vi "rad_Configure Target Dialog.vi"(8 "Error In":errorcluster, 11 "Target Information in":T1={"Hostname"="", "Serial number"="", "Product name"="", "Product code"=0, "System status"="", "Credential type"=enum."None/Unlocked", "User added?"=FALSE, "Primary NIC"={"MAC address"="", "IP Address Request Mode"=2, "IP address"="", "Subnet mask"="", "Gateway"="", "DNS server"=""}, "System Credentials"={"Username"="", "Password"=""}} {"Primary NIC"."IP Address Request Mode" items=["Static"=1, "DHCP/Link-Local"=2, "Link-Local Only"=4, "DHCP Only"=8]}) -> (0 "Error Out":errorcluster, 3 "Target Information out":T1={"Hostname"="", "Serial number"="", "Product name"="", "Product code"=0, "System status"="", "Credential type"=enum."None/Unlocked", "User added?"=FALSE, "Primary NIC"={"MAC address"="", "IP Address Request Mode"=2, "IP address"="", "Subnet mask"="", "Gateway"="", "DNS server"=""}, "System Credentials"={"Username"="", "Password"=""}} {"Primary NIC"."IP Address Request Mode" items=["Static"=1, "DHCP/Link-Local"=2, "Link-Local Only"=4, "DHCP Only"=8]})   [LabVIEW 2020]
uses:
  support/SubVIs/Target Information.ctl
  TypeDefs/rad_Target Network Settings.ctl
  support/SubVIs/System Credentials.ctl
panel:
  in  "IP Address Request Mode":i32(ring)=2 items=["Static"=1, "DHCP/Link-Local"=2, "Link-Local Only"=4, "DHCP Only"=8]
  in  "DNS":string
  in  "Gateway":string
  in  "Subnet Mask":string
  in  "IP Address":string
  in  "Host Name":string
  in  "Cancel":bool
  in  "OK":bool
  # "Network Configuration"
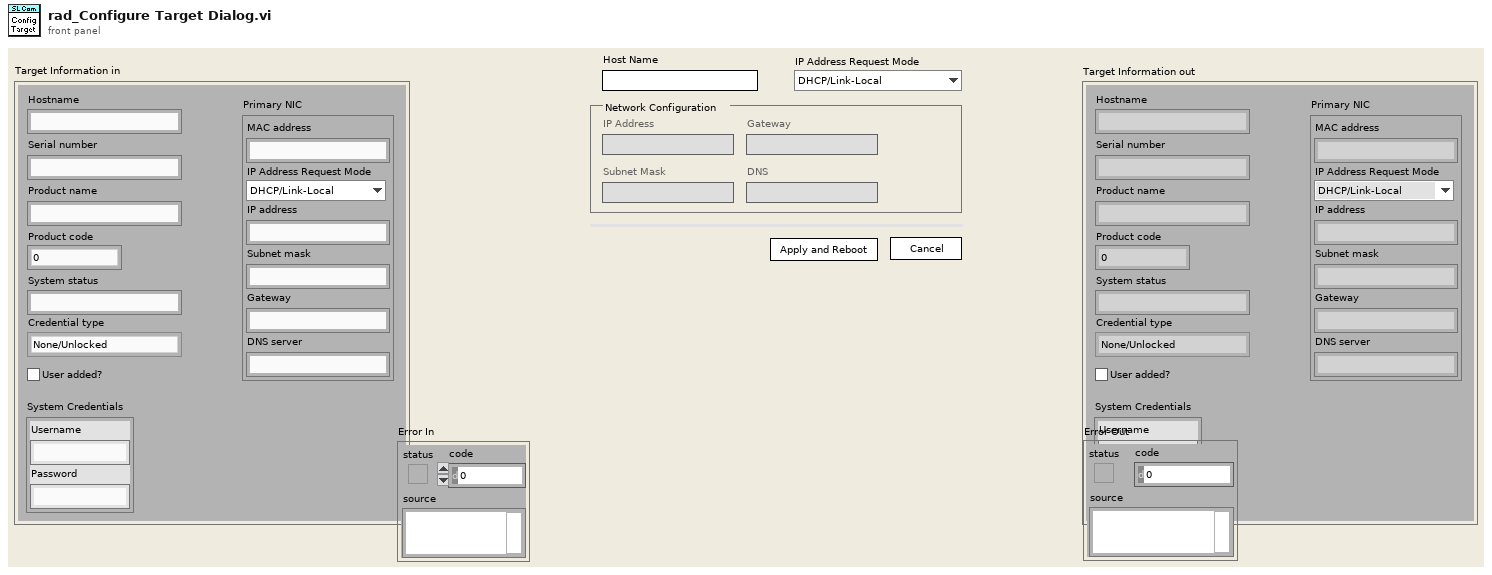
[diagram p1: front panel]
types:
  T1 = typedef "Target Information.ctl" = cluster{"Hostname":string, "Serial number":string, "Product name":string, "Product code":i32, "System status":string, "Credential type":enum16{"None/Unlocked", "FTP Password", "NIAuth Credentials"}, "User added?":bool, "Primary NIC":T2, "System Credentials":T3}
  T2 = typedef "rad_Target Network Settings.ctl" = cluster{"MAC address":string, "IP Address Request Mode":i32, "IP address":string, "Subnet mask":string, "Gateway":string, "DNS server":string}
  T3 = typedef "System Credentials.ctl" = cluster{"Username":string, "Password":string}
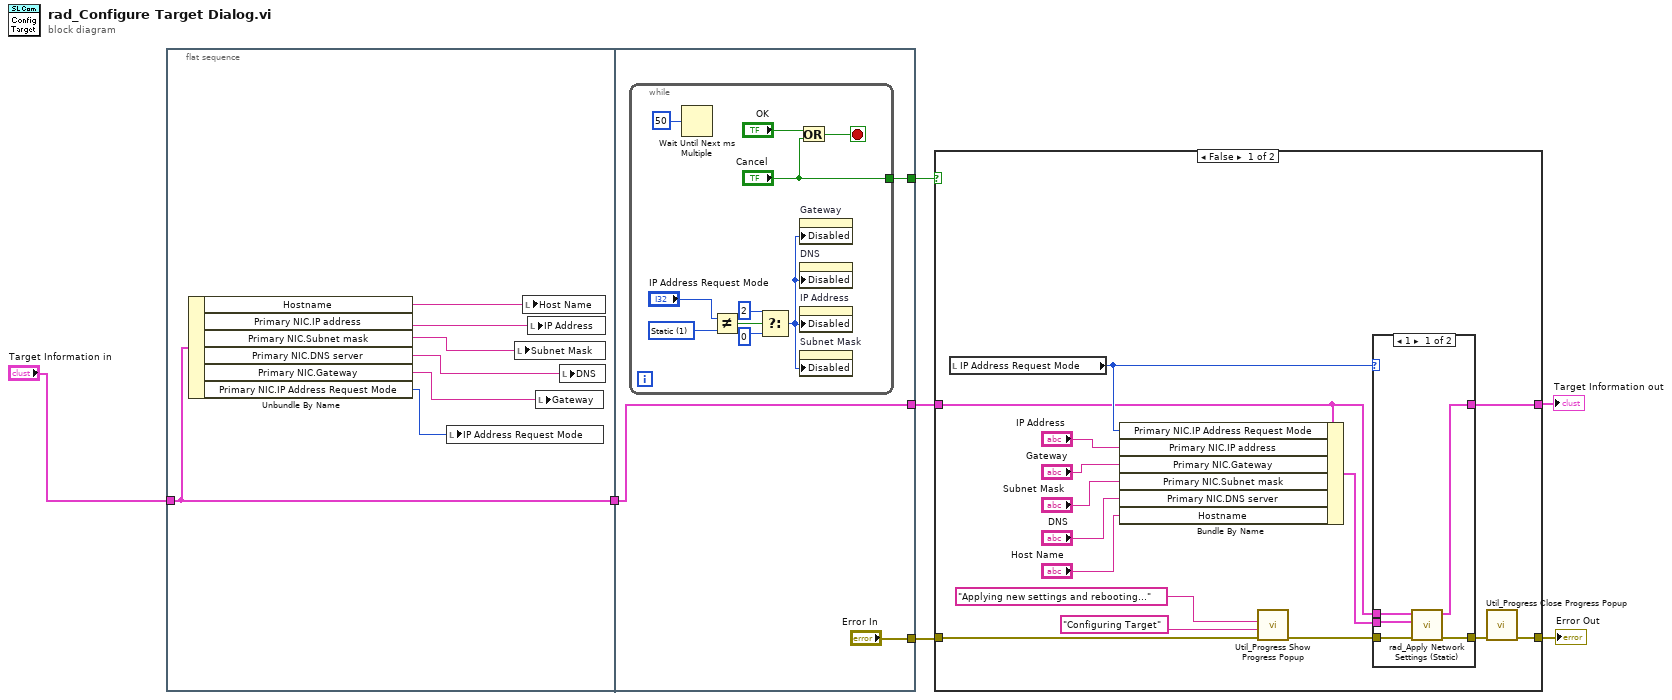
[diagram p0: block diagram]
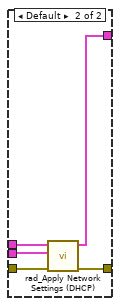
[diagram p2: hidden frame]
diagram:
  n1 = flat-sequence {
    tunnel: "Target Information in" -> [w8]
    tunnel: [w8] -> w1
    tunnel: [w17] -> w5
    tunnel: [w15] -> w4
    tunnel: ["Error In"] -> w3
    tunnel: w1 -> [w15]
    frame #0 {
      n2 = Unbundle By Name(w8) -> ("Hostname"=w14:string, "Primary NIC.IP address"=w13:string, "Primary NIC.Subnet mask"=w12:string, "Primary NIC.DNS server"=w11:string, "Primary NIC.Gateway"=w10:string, "Primary NIC.IP Address Request Mode"=w9:i32)
      n3 = local write "IP Address Request Mode"(w9) -> ()
      n4 = local write "Subnet Mask"(w12) -> ()
      n5 = local write "Host Name"(w14) -> ()
      n6 = local write "IP Address"(w13) -> ()
      n7 = local write "Gateway"(w10) -> ()
      n8 = local write "DNS"(w11) -> ()
    }
    frame #1 {
      n9 = while {
        tunnel: ["Cancel"] -> w17
        stop <- w25 stop-if-true
        w19 = 1 items=["Static"=1, "DHCP/Link-Local"=2, "Link-Local Only"=4, "DHCP Only"=8] ("IP Address Request Mode")
        n10 = Wait Until Next ms Multiple(millisecond multiple=u32 50) -> ()  [unwired: 1 out]
        n11 = Not Equal?(x="IP Address Request Mode", y=w19) -> (x != y?=w18:bool)
        n12 = Select(t=u8 2 ("Disabled"), s=w18, f=u8 0 ("Disabled")) -> (s? t:f=w21:u8)
        n13 = Or(x="OK", y="Cancel") -> (x .or. y?=w25:bool)
        n14 = property on="Gateway" class="Str"("Disabled"=w21) -> ()  [unwired: 2 in, 2 out]
        n15 = property on="DNS" class="Str"("Disabled"=w21) -> ()  [unwired: 2 in, 2 out]
        n16 = property on="IP Address" class="Str"("Disabled"=w21) -> ()  [unwired: 2 in, 2 out]
        n17 = property on="Subnet Mask" class="Str"("Disabled"=w21) -> ()  [unwired: 2 in, 2 out]
      }
    }
  }
  n18 = case shown="False" w5 {
    tunnel: w4 -> [w28 w54]
    tunnel: [w29 w54] -> w6
    tunnel: [w37 w53] -> w7
    tunnel: w3 -> [w40 w53]
    frame False {
      n19 = local read "IP Address Request Mode"() -> (w32:i32)
      n20 = Bundle By Name(cluster=w28, "Primary NIC.IP Address Request Mode"=w32, "Primary NIC.IP address"="IP Address", "Primary NIC.Gateway"="Gateway", "Primary NIC.Subnet mask"="Subnet Mask", "Primary NIC.DNS server"="DNS", "Hostname"="Host Name") -> (w31:T1)
      n21 = call "Util_Progress Show Progress Popup.vi"("error in (no error)"=w40, "Title"="Configuring Target", "Message"="Applying new settings and rebooting...") -> ("error out"=w38:errorcluster)  [unwired: 1 in, 7 out]
      n22 = case shown="1" w32 {
        tunnel: [w46 w51] -> w39
        tunnel: w38 -> [w47 w52]
        tunnel: w31 -> [w44 w49]
        tunnel: [w43 w50] -> w29
        tunnel: w28 -> [w45 w48]
        frame 1 {
          n23 = call "rad_Apply Network Settings (Static).vi"("error in (no error)"=w47, "Requested settings"=w44, "Existing settings"=w45) -> ("error out"=w46:errorcluster, "Target settings out"=w43:T1)  [unwired: 7 in]
        }
        frame Default {
          n24 = call "rad_Apply Network Settings (DHCP).vi"("error in (no error)"=w52, "Requested settings"=w49, "Existing settings"=w48) -> ("error out"=w51:errorcluster, "Target settings out"=w50:T1)  [unwired: 7 in]
        }
      }
      n25 = call "Util_Progress Close Progress Popup.vi"("error in (no error)"=w39) -> ("error out"=w37:errorcluster)  [unwired: 2 in, 8 out]
    }
    frame True {
    }
  }
  "Target Information out" <- w6
  "Error Out" <- w7
